vi "Get Page VI.vi"(8 "error in":errorcluster, 9 "GUID":string, 10 "item ref":T1 format="%.0x", 11 "System Explorer Dispatcher Implementation in":refnum<class "System Explorer Dispatcher.lvclass">) -> (0 "error out":errorcluster, 2 "page reference":refnum<vi>, 3 "System Explorer Dispatcher Implementation out":refnum<class "System Explorer Dispatcher.lvclass">)   [LabVIEW 2020, in "AIM MIL-STD-1553 System Explorer.lvlib" / "Implementation.lvlib" / "System Explorer Dispatcher.lvclass"]
uses:
  System Explorer Dispatcher.lvclass
  <vilib>/NI VeriStand/Custom Device API/Custom Device Item Ref.ctl
  <vilib>/NI VeriStand/Custom Device API/Custom Device API.lvlib
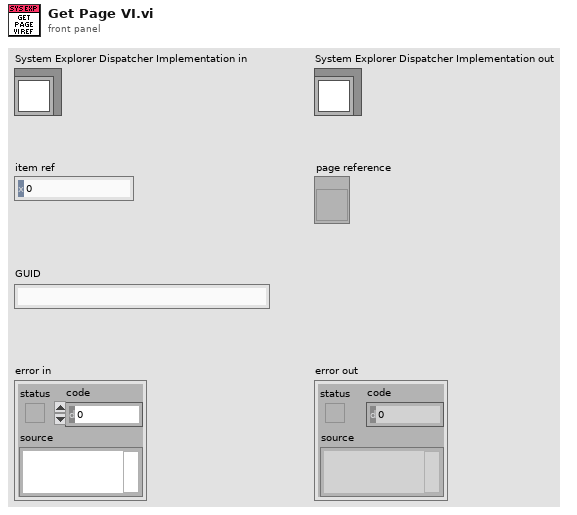
[diagram p1: front panel]
types:
  T1 = typedef "Custom Device API.lvlib/Custom Device Item Ref.ctl" = u64
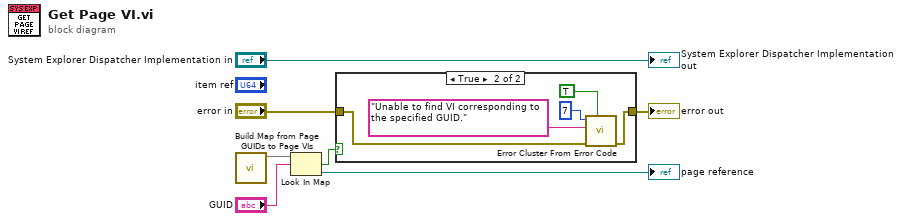
[diagram p0: block diagram]
diagram:
  n1 = call "Build Map from Page GUIDs to Page VIs.vi"() -> ("page map GUID to VI ref"=w6:map{string, refnum<vi>})  [unwired: 11 in]
  n2 = Look In Map(map=w6, key="GUID") -> (key not found?=w4:bool, value=→"page reference":refnum<vi>)  [unwired: 1 in]
  n3 = case shown="True" w4 {
    tunnel: [w8 w10] -> w3
    tunnel: "error in" -> [w8 w9]
    frame False {
    }
    frame True {
      n4 = call <vilib>:"Error Cluster From Error Code.vi"("show call chain? (False)"=TRUE, "error in (no error)"=w9, "error message (\"\")"="Unable to find VI corresponding to the specified GUID." ("error message (\"\")"), "error code (0)"=7) -> ("error out"=w10:errorcluster)  [unwired: 5 in]
    }
  }
  "error out" <- w3
  "System Explorer Dispatcher Implementation out" <- "System Explorer Dispatcher Implementation in"
